vi "demo.vi"() -> ()   [LabVIEW 2022 SP3]
uses:
  Components/ViPER.lvlibp/ViPER.lvclass
panel:
  in  "String":string="<?xml version=\"1.0\" encoding=\"UTF-8\" standalone=\"no\" ?>\n<Object>\n\n  <Name>Matrix_1</Name>\n\n  <Class>Switch_Keysight_34934A</Class>\n\n  <Config>\n    <NumElts>4</NumElts>\n    <Refnum>\n      <Name>VISA</Name>\n      <RefKind>VISA</RefKind>\n      <Val>USB0::0x0957::0x0507::MY56485422::INSTR</Val>\n</Refnum>\n    <I32>\n      <Name>Slot</Name>\n      <Val>1</Val>\n</I32>\n    <Array>\n      <Name>SwitchMap</Name>\n      <Dimsize>11</Dimsize>\n      <Cluster>\n        <Name>Alias</Name>\n        <NumElts>7</NumElts>\n        <String>\n          <Name>Name</Name>\n          <Val>PassiveTests</Val>\n</String>\n        <Array>\n          <Name>Route</Name>\n          <Dimsize>0</Dimsize>\n          <String>\n            <Name>String</Name>\n            <Val/>\n</String>\n</Array>\n        <Array>\n          <Name>UnRoute</Name>\n          <Dimsize>0</Dimsize>\n          <String>\n            <Name>String</Name>\n            <Val/>\n</String>\n</Array>\n        <String>\n          <Name>Description</Name>\n          <Val>Tests component values unpowered</Val>\n</String>\n        <String>\n          <Name>Dependancies</Name>\n          <Val/>\n</String>\n        <String>\n          <Name>Group</Name>\n          <Val/>\n</String>\n        <Boolean>\n          <Name>IsGroup</Name>\n          <Val>1</Val>\n</Boolean>\n</Cluster>\n      <Cluster>\n        <Name>Alias</Name>\n        <NumElts>7</NumElts>\n        <String>\n          <Name>Name</Name>\n          <Val>Discharge_C108_C109</Val>\n</String>\n        <Array>\n          <Name>Route</Name>\n          <Dimsize>4</Dimsize>\n          <String>\n            <Name>String</Name>\n            <Val>M1H:1:6:1</Val>\n</String>\n          <String>\n            <Name>String</Name>\n            <Val>M1H:1:19:1</Val>\n</String>\n          <String>\n            <Name>String</Name>\n            <Val>M1L:1:6:1</Val>\n</String>\n          <String>\n            <Name>String</Name>\n            <Val>M1L:1:19:1</Val>\n</String>\n</Array>\n        <Array>\n          <Name>UnRoute</Name>\n          <Dimsize>4</Dimsize>\n          <String>\n            <Name>String</Name>\n            <Val>M1H:1:6:0</Val>\n</String>\n          <String>\n            <Name>String</Name>\n            <Val>M1H:1:19:0</Val>\n</String>\n          <String>\n            <Name>String</Name>\n            <Val>M1L:1:6:0</Val>\n</String>\n          <String>\n            <Name>String</Name>\n            <Val>M1L:1:19:0</Val>\n</String>\n</Array>\n        <String>\n          <Name>Description</Name>\n          <Val>Discharge the caps for 3 secs</Val>\n</String>\n        <String>\n          <Name>Dependancies</Name>\n          <Val/>\n</String>\n        <String>\n          <Name>Group</Name>\n          <Val>PassiveTests</Val>\n</String>\n        <Boolean>\n          <Name>IsGroup</Name>\n          <Val>0</Val>\n</Boolean>\n</Cluster>\n      <Cluster>\n        <Name>Alias</Name>\n        <NumElts>7</NumElts>\n        <String>\n          <Name>Name</Name>\n          <Val>CapacitorTests</Val>\n</String>\n        <Array>\n          <Name>Route</Name>\n          <Dimsize>0</Dimsize>\n          <String>\n            <Name>String</Name>\n            <Val/>\n</String>\n</Array>\n        <Array>\n          <Name>UnRoute</Name>\n          <Dimsize>0</Dimsize>\n          <String>\n            <Name>String</Name>\n            <Val/>\n</String>\n</Array>\n        <String>\n          <Name>Description</Name>\n          <Val>Tests Capacitor Values</Val>\n</String>\n        <String>\n          <Name>Dependancies</Name>\n          <Val/>\n</String>\n        <String>\n          <Name>Group</Name>\n          <Val>PassiveTests</Val>\n</String>\n        <Boolean>\n          <Name>IsGroup</Name>\n          <Val>1</Val>\n</Boolean>\n</Cluster>\n      <Cluster>\n        <Name>Alias</Name>\n        <NumElts>7</NumElts>\n        <String>\n          <Name>Name</Name>\n          <Val>Connect_LCR</Val>\n</String>\n        <Array>\n          <Name>Route</Name>\n          <Dimsize>4</Dimsize>\n          <String>\n            <Name>String</Name>\n            <Val>M1H:1:23:1</Val>\n</String>\n          <String>\n            <Name>String</Name>\n            <Val>M1H:2:24:1</Val>\n</String>\n          <String>\n            <Name>String</Name>\n            <Val>M1L:1:25:1</Val>\n</String>\n          <String>\n            <Name>String</Name>\n            <Val>M1L:2:26:1</Val>\n</String>\n</Array>\n        <Array>\n          <Name>UnRoute</Name>\n          <Dimsize>4</Dimsize>\n          <String>\n            <Name>String</Name>\n            <Val>M1H:1:23:0</Val>\n</String>\n          <String>\n            <Name>String</Name>\n            <Val>M1H:2:24:0</Val>\n</String>\n          <String>\n            <Name>String</Name>\n            <Val>M1L:1:25:0</Val>\n</String>\n          <String>\n            <Name>String</Name>\n            <Val>M1L:2:26:0</Val>\n</String>\n</Array>\n        <String>\n          <Name>Description</Name>\n          <Val>Connect the LCR to the Matrix</Val>\n</String>\n        <String>\n          <Name>Dependancies</Name>\n          <Val>Discharge_C108_C109</Val>\n</String>\n        <String>\n          <Name>Group</Name>\n          <Val>CapacitorTests</Val>\n</String>\n        <Boolean>\n          <Name>IsGroup</Name>\n          <Val>0</Val>\n</Boolean>\n</Cluster>\n      <Cluster>\n        <Name>Alias</Name>\n        <NumElts>7</NumElts>\n        <String>\n          <Name>Name</Name>\n          <Val>C108_C109</Val>\n</String>\n        <Array>\n          <Name>Route</Name>\n          <Dimsize>4</Dimsize>\n          <String>\n            <Name>String</Name>\n            <Val>M1H:1:6:1</Val>\n</String>\n          <String>\n            <Name>String</Name>\n            <Val>M1H:2:6:1</Val>\n</String>\n          <String>\n            <Name>String</Name>\n            <Val>M1L:1:6:1</Val>\n</String>\n          <String>\n            <Name>String</Name>\n            <Val>M1L:2:6:1</Val>\n</String>\n</Array>\n        <Array>\n          <Name>UnRoute</Name>\n          <Dimsize>4</Dimsize>\n          <String>\n            <Name>String</Name>\n            <Val>M1H:1:6:0</Val>\n</String>\n          <String>\n            <Name>String</Name>\n            <Val>M1H:2:6:0</Val>\n</String>\n          <String>\n            <Name>String</Name>\n            <Val>M1L:1:6:0</Val>\n</String>\n          <String>\n            <Name>String</Name>\n            <Val>M1L:2:6:0</Val>\n</String>\n</Array>\n        <String>\n          <Name>Description</Name>\n          <Val>C108 and C109 to LCR</Val>\n</String>\n        <String>\n          <Name>Dependancies</Name>\n          <Val>Discharge_C108_C109, Connect_LCR</Val>\n</String>\n        <String>\n          <Name>Group</Name>\n          <Val>CapacitorTests</Val>\n</String>\n        <Boolean>\n          <Name>IsGroup</Name>\n          <Val>0</Val>\n</Boolean>\n</Cluster>\n      <Cluster>\n        <Name>Alias</Name>\n        <NumElts>7</NumElts>\n        <String>\n          <Name>Name</Name>\n          <Val>C153</Val>\n</String>\n        <Array>\n          <Name>Route</Name>\n          <Dimsize>4</Dimsize>\n          <String>\n            <Name>String</Name>\n            <Val>M1H:1:7:1</Val>\n</String>\n          <String>\n            <Name>String</Name>\n            <Val>M1H:2:7:1</Val>\n</String>\n          <String>\n            <Name>String</Name>\n            <Val>M1L:1:5:1</Val>\n</String>\n          <String>\n            <Name>String</Name>\n            <Val>M1L:2:5:1</Val>\n</String>\n</Array>\n        <Array>\n          <Name>UnRoute</Name>\n          <Dimsize>4</Dimsize>\n          <String>\n            <Name>String</Name>\n            <Val>M1H:1:7:0</Val>\n</String>\n          <String>\n            <Name>String</Name>\n            <Val>M1H:2:7:0</Val>\n</String>\n          <String>\n            <Name>String</Name>\n            <Val>M1L:1:5:0</Val>\n</String>\n          <String>\n            <Name>String</Name>\n            <Val>M1L:2:5:0</Val>\n</String>\n</Array>\n        <String>\n          <Name>Description</Name>\n          <Val>C153 to LCR</Val>\n</String>\n        <String>\n          <Name>Dependancies</Name>\n          <Val>Discharge_C108_C109, Connect_LCR</Val>\n</String>\n        <String>\n          <Name>Group</Name>\n          <Val>CapacitorTests</Val>\n</String>\n        <Boolean>\n          <Name>IsGroup</Name>\n          <Val>0</Val>\n</Boolean>\n</Cluster>\n      <Cluster>\n        <Name>Alias</Name>\n        <NumElts>7</NumElts>\n        <String>\n          <Name>Name</Name>\n          <Val>C1300</Val>\n</String>\n        <Array>\n          <Name>Route</Name>\n          <Dimsize>4</Dimsize>\n          <String>\n            <Name>String</Name>\n            <Val>M1H:1:2:1</Val>\n</String>\n          <String>\n            <Name>String</Name>\n            <Val>M1H:2:2:1</Val>\n</String>\n          <String>\n            <Name>String</Name>\n            <Val>M1L:1:7:1</Val>\n</String>\n          <String>\n            <Name>String</Name>\n            <Val>M1L:2:7:1</Val>\n</String>\n</Array>\n        <Array>\n          <Name>UnRoute</Name>\n          <Dimsize>4</Dimsize>\n          <String>\n            <Name>String</Name>\n            <Val>M1H:1:2:0</Val>\n</String>\n          <String>\n            <Name>String</Name>\n            <Val>M1H:2:2:0</Val>\n</String>\n          <String>\n            <Name>String</Name>\n            <Val>M1L:1:7:0</Val>\n</String>\n          <String>\n            <Name>String</Name>\n            <Val>M1L:2:7:0</Val>\n</String>\n</Array>\n        <String>\n          <Name>Description</Name>\n          <Val>C1300 to LCR</Val>\n</String>\n        <String>\n          <Name>Dependancies</Name>\n          <Val>Discharge_C108_C109, Connect_LCR</Val>\n</String>\n        <String>\n          <Name>Group</Name>\n          <Val>CapacitorTests</Val>\n</String>\n        <Boolean>\n          <Name>IsGroup</Name>\n          <Val>0</Val>\n</Boolean>\n</Cluster>\n      <Cluster>\n        <Name>Alias</Name>\n        <NumElts>7</NumElts>\n        <String>\n          <Name>Name</Name>\n          <Val>C701</Val>\n</String>\n        <Array>\n          <Name>Route</Name>\n          <Dimsize>4</Dimsize>\n          <String>\n            <Name>String</Name>\n            <Val>M1H:1:8:1</Val>\n</String>\n          <String>\n            <Name>String</Name>\n            <Val>M1H:2:8:1</Val>\n</String>\n          <String>\n            <Name>String</Name>\n            <Val>M1L:1:2:1</Val>\n</String>\n          <String>\n            <Name>String</Name>\n            <Val>M1L:2:2:1</Val>\n</String>\n</Array>\n        <Array>\n          <Name>UnRoute</Name>\n          <Dimsize>4</Dimsize>\n          <String>\n            <Name>String</Name>\n            <Val>M1H:1:8:0</Val>\n</String>\n          <String>\n            <Name>String</Name>\n            <Val>M1H:2:8:0</Val>\n</String>\n          <String>\n            <Name>String</Name>\n            <Val>M1L:1:2:0</Val>\n</String>\n          <String>\n            <Name>String</Name>\n            <Val>M1L:2:2:0</Val>\n</String>\n</Array>\n        <String>\n          <Name>Description</Name>\n          <Val>C701 to LCR</Val>\n</String>\n        <String>\n          <Name>Dependancies</Name>\n          <Val>Discharge_C108_C109, Connect_LCR</Val>\n</String>\n        <String>\n          <Name>Group</Name>\n          <Val>CapacitorTests</Val>\n</String>\n        <Boolean>\n          <Name>IsGroup</Name>\n          <Val>0</Val>\n</Boolean>\n</Cluster>\n      <Cluster>\n        <Name>Alias</Name>\n        <NumElts>7</NumElts>\n        <String>\n          <Name>Name</Name>\n          <Val>C1202</Val>\n</String>\n        <Array>\n          <Name>Route</Name>\n          <Dimsize>4</Dimsize>\n          <String>\n            <Name>String</Name>\n            <Val>M1H:1:2:1</Val>\n</String>\n          <String>\n            <Name>String</Name>\n            <Val>M1H:2:2:1</Val>\n</String>\n          <String>\n            <Name>String</Name>\n            <Val>M1L:1:8:1</Val>\n</String>\n          <String>\n            <Name>String</Name>\n            <Val>M1L:2:8:1</Val>\n</String>\n</Array>\n        <Array>\n          <Name>UnRoute</Name>\n          <Dimsize>4</Dimsize>\n          <String>\n            <Name>String</Name>\n            <Val>M1H:1:2:0</Val>\n</String>\n          <String>\n            <Name>String</Name>\n            <Val>M1H:2:2:0</Val>\n</String>\n          <String>\n            <Name>String</Name>\n            <Val>M1L:1:8:0</Val>\n</String>\n          <String>\n            <Name>String</Name>\n            <Val>M1L:2:8:0</Val>\n</String>\n</Array>\n        <String>\n          <Name>Description</Name>\n          <Val>C1202 to LCR</Val>\n</String>\n        <String>\n          <Name>Dependancies</Name>\n          <Val>Discharge_C108_C109, Connect_LCR</Val>\n</String>\n        <String>\n          <Name>Group</Name>\n          <Val>CapacitorTests</Val>\n</String>\n        <Boolean>\n          <Name>IsGroup</Name>\n          <Val>0</Val>\n</Boolean>\n</Cluster>\n      <Cluster>\n        <Name>Alias</Name>\n        <NumElts>7</NumElts>\n        <String>\n          <Name>Name</Name>\n          <Val>C1204</Val>\n</String>\n        <Array>\n          <Name>Route</Name>\n          <Dimsize>4</Dimsize>\n          <String>\n            <Name>String</Name>\n            <Val>M1H:1:9:1</Val>\n</String>\n          <String>\n            <Name>String</Name>\n            <Val>M1H:2:9:1</Val>\n</String>\n          <String>\n            <Name>String</Name>\n            <Val>M1L:1:2:1</Val>\n</String>\n          <String>\n            <Name>String</Name>\n            <Val>M1L:2:2:1</Val>\n</String>\n</Array>\n        <Array>\n          <Name>UnRoute</Name>\n          <Dimsize>4</Dimsize>\n          <String>\n            <Name>String</Name>\n            <Val>M1H:1:9:0</Val>\n</String>\n          <String>\n            <Name>String</Name>\n            <Val>M1H:2:9:0</Val>\n</String>\n          <String>\n            <Name>String</Name>\n            <Val>M1L:1:2:0</Val>\n</String>\n          <String>\n            <Name>String</Name>\n            <Val>M1L:2:2:0</Val>\n</String>\n</Array>\n        <String>\n          <Name>Description</Name>\n          <Val>C1204 to LCR</Val>\n</String>\n        <String>\n          <Name>Dependancies</Name>\n          <Val>Discharge_C108_C109, Connect_LCR</Val>\n</String>\n        <String>\n          <Name>Group</Name>\n          <Val>CapacitorTests</Val>\n</String>\n        <Boolean>\n          <Name>IsGroup</Name>\n          <Val>0</Val>\n</Boolean>\n</Cluster>\n      <Cluster>\n        <Name>Alias</Name>\n        <NumElts>7</NumElts>\n        <String>\n          <Name>Name</Name>\n          <Val>C1200</Val>\n</String>\n        <Array>\n          <Name>Route</Name>\n          <Dimsize>4</Dimsize>\n          <String>\n            <Name>String</Name>\n            <Val>M1H:1:2:1</Val>\n</String>\n          <String>\n            <Name>String</Name>\n            <Val>M1H:2:2:1</Val>\n</String>\n          <String>\n            <Name>String</Name>\n            <Val>M1L:1:9:1</Val>\n</String>\n          <String>\n            <Name>String</Name>\n            <Val>M1L:2:9:1</Val>\n</String>\n</Array>\n        <Array>\n          <Name>UnRoute</Name>\n          <Dimsize>4</Dimsize>\n          <String>\n            <Name>String</Name>\n            <Val>M1H:1:2:0</Val>\n</String>\n          <String>\n            <Name>String</Name>\n            <Val>M1H:2:2:0</Val>\n</String>\n          <String>\n            <Name>String</Name>\n            <Val>M1L:1:9:0</Val>\n</String>\n          <String>\n            <Name>String</Name>\n            <Val>M1L:2:9:0</Val>\n</String>\n</Array>\n        <String>\n          <Name>Description</Name>\n          <Val>C1200 to LCR</Val>\n</String>\n        <String>\n          <Name>Dependancies</Name>\n          <Val>Discharge_C108_C109, Connect_LCR</Val>\n</String>\n        <String>\n          <Name>Group</Name>\n          <Val>CapacitorTests</Val>\n</String>\n        <Boolean>\n          <Name>IsGroup</Name>\n          <Val>0</Val>\n</Boolean>\n</Cluster>\n</Array>\n    <Boolean>\n      <Name>Sim</Name>\n      <Val>1</Val>\n</Boolean>\n</Config>  <Ancestors>\n    <Ancestor>\n      <Class>SwitchBase</Class>\n      <Config>\n        <NumElts>1</NumElts>\n        <String>\n          <Name>default</Name>\n          <Val/>\n</String>\n</Config>    </Ancestor>\n  </Ancestors>\n\n</Object>\n"
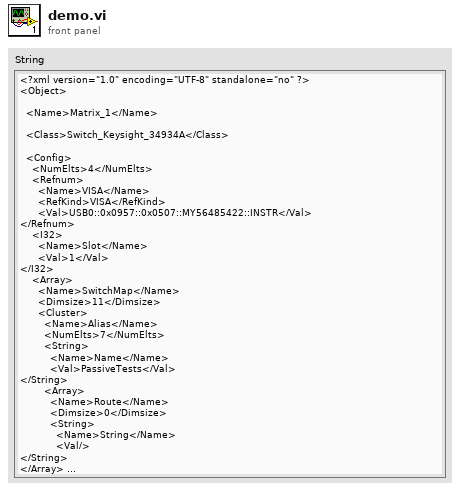
[diagram p1: front panel]
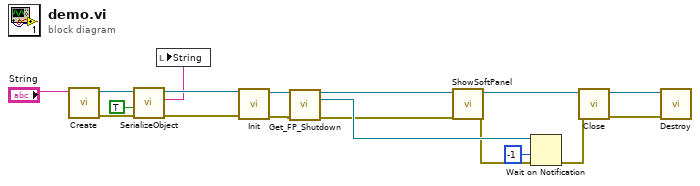
[diagram p0: block diagram]
diagram:
  n1 = call "Create.vi"("Config XML"="String") -> ("error out"=w8:errorcluster, "reference out"=w6:refnum<class "ViPER.lvclass">)  [unwired: 9 in]
  n2 = call-dynamic "SerializeObject.vi"("error in (no error)"=w8, "Pretty Print?"=TRUE, "ViPER_Base in"=w6) -> ("error out"=w7:errorcluster, "Object XML"=w3:string, "ViPER_Base out"=w5:refnum<class "ViPER.lvclass">)  [unwired: 6 in]
  n3 = local write "String"(w3) -> ()
  n4 = call-dynamic "Init.vi"("error in (no error)"=w7, "reference in"=w5) -> ("error out"=w16:errorcluster, "reference out"=w17:refnum<class "ViPER.lvclass">)  [unwired: 8 in]
  n5 = call "Get_FP_Shutdown.vi"("ViPER_Base in"=w17, "error in (no error)"=w16) -> ("ViPER_Base out"=w1:refnum<class "ViPER.lvclass">, "SoftFP_Shutdown"=w15:refnum<notifier>, "error out"=w2:errorcluster)  [unwired: 10 in, 1 out]
  n6 = call-dynamic "ShowSoftPanel.vi"("error in (no error)"=w2, "Driver in"=w1) -> ("error out"=w14:errorcluster, "Driver out"=w11:refnum<class "ViPER.lvclass">)  [unwired: 7 in, 1 out]
  n7 = Wait on Notification(notifier=w15, timeout in ms (-1)=-1, error in (no error)=w14) -> (error out=w12:errorcluster)  [unwired: 1 in, 3 out]
  n8 = call-dynamic "Close.vi"("error in (no error)"=w12, "reference in"=w11) -> ("error out"=w10:errorcluster, "reference out"=w9:refnum<class "ViPER.lvclass">)  [unwired: 8 in]
  n9 = call "Destroy.vi"("error in (no error)"=w10, "reference in"=w9) -> ()  [unwired: 9 in, 1 out]
